vi "Analyze.vi"(8 "error in (no error)":errorcluster, 10 "Image in":T1, 11 "Analyze Q-Factor in":refnum<class "Analyze q-Factor.lvclass">) -> (0 "error out":errorcluster, 1 "Results":refnum<class "Analyze Results Base.lvclass">, 2 "Image out":T1, 3 "Analyze Q-Factor out":refnum<class "Analyze q-Factor.lvclass">)   [LabVIEW 2020, in "Analyze.lvlib" / "Analyze q-Factor.lvclass"]
uses:
  Analyze q-Factor.lvclass
  C:/POLARIS Programme/POLARIS-AS-3-Cams/Submodules/HIJ Vision/Analyze/Analyze Classes/Analyze BaseClass/Analyze BaseClass/Analyze BaseClass.lvclass
  <vilib>/vision/Image Controls.llb/IMAQ Image.ctl
  Results and Overlays/Results Base/Analyze Results Base.lvclass
  Results and Overlays/Results q-Factor/Analyze Results q-Factor.lvclass
  C:/POLARIS Programme/POLARIS-AS-3-Cams/Submodules/HIJ Vision/Analyze/Results and Overlays/Results Base/Analyze Results Base.lvclass
  Results and Overlays/Results Fluence/Analyze Results Fluence.lvclass
  Analyze Parameter/Analyze Parameter Width Method/Width Method.lvclass
  C:/POLARIS Programme/POLARIS-AS-3-Cams/Submodules/HIJ Vision/Analyze/Analyze Parameter/Analyze Parameter Base/Analyze Parameter Base.lvclass
  Results and Overlays/Results q-Factor/Analyze Results q-Factor.lvclass/Analyze Results q-Factor.ctl
  Results and Overlays/Results q-Factor/Write A.vi
  Results and Overlays/Results q-Factor/Write q.vi
  Results and Overlays/Results q-Factor/Write Focus ROI.vi
  Results and Overlays/Results q-Factor/Write Width Method.vi
  Analyze Fluence/Analyze Fluence.lvclass
  <vilib>/vision/NI_Vision_Development_Module.lvlib
  Analyze BaseClass/Analyze BaseClass/Analyze BaseClass.lvclass
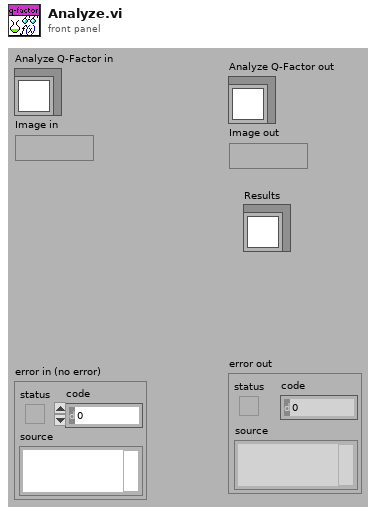
[diagram p1: front panel]
types:
  T1 = typedef "IMAQ Image.ctl" = refnum<image>
  T2 = typedef "Image Type" = u32
  T3 = typedef "Analyze.lvlib/Analyze Fluence.lvclass/Fluence Info.ctl" = cluster{"Fluence J/cm^2":dbl[unit], "Energy in Area":dbl[unit], "max value":i64, "Max fluence area":cluster{"Left":i32, "Top":i32, "Right":i32, "Bottom":i32}}
  T4 = cluster{"Left":i32, "Top":i32, "Right":i32, "Bottom":i32, sgl}
  T5 = typedef "ROI Descriptor" = cluster{"Global Rectangle":i32[], "Contours":cluster{"ID":enum32{"External", "Internal"}, "Type":u32, "Coordinates":i32[]}[]}
  T6 = typedef "POLARIS Vision utility.lvlib/Width Method.ctl" = enum16{"FWHM", "1/e", "1/e^2", "80%", "90%"}
  T7 = cluster{"Mean Value":sgl, "Standard Variation":sgl, "Minimal Value":sgl, "Maximal Value":sgl, "Area (calibrated)":sgl, "Area (pixels)":i32, "%":sgl}
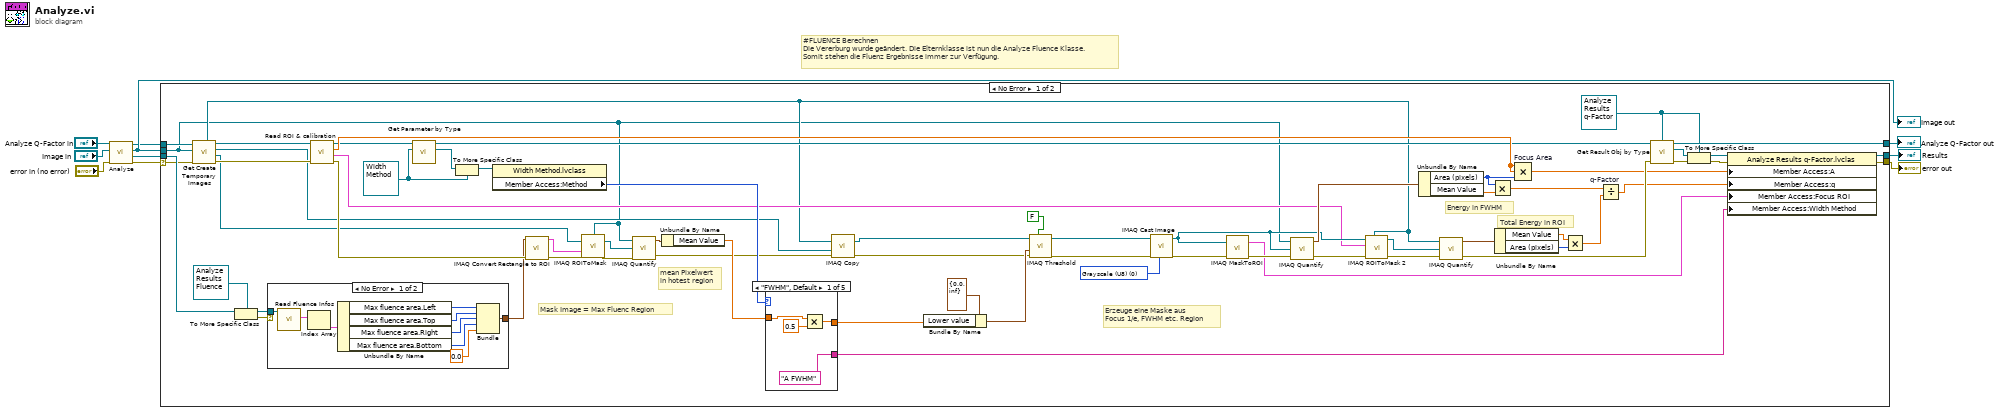
[diagram p0: block diagram]
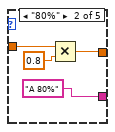
[diagram p3: hidden frame]
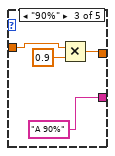
[diagram p4: hidden frame]
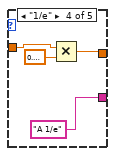
[diagram p5: hidden frame]
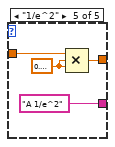
[diagram p6: hidden frame]
diagram:
  # "#FLUENCE Berechnen\nDie Vererburg wurde geändert. Die Elternklasse ist nun die Analyze Fluence Klasse.\nSomit stehen die Fluenz Ergebnisse immer zur Verfügung."
  n1 = call-parent "Analyze.vi"("error in (no error)"="error in (no error)", "Image in"="Image in", "Analyze Fluence in"="Analyze Q-Factor in") -> ("error out"=w2:errorcluster, "Result"=w4:refnum<class "Analyze Results Base.lvclass">, "Image out"=w10:T1, "Analyze Fluence out"=w6:refnum<class "Analyze q-Factor.lvclass">)  [unwired: 5 in]
  "Image out" <- w10
  n2 = case shown="No Error" w2 {
    selector: w2 -> [w21 w106]
    tunnel: w10 -> [w11 _]
    tunnel: w6 -> [w49 w107]
    tunnel: [w44 w105] -> w5
    tunnel: w4 -> [w36 w105]
    tunnel: [w27 w107] -> w3
    tunnel: [w43 w106] -> w1
    frame No Error {
      w29 = refnum<class "Width Method.lvclass"> refnum ("Width Method.lvclass")
      w24 = refnum<class "Analyze Results q-Factor.lvclass"> refnum ("Analyze Results q-Factor.lvclass")
      w70 = T2 0 items=["Grayscale (U8)", "Grayscale (I16)", "Grayscale (SGL)", "Complex (CSG)", "RGB (U32)", "HSL (U32)", "RGB (U64)", "Grayscale (U16)"] ("Image Type")
      # "Erzeuge eine Maske aus \nFocus 1/e, FWHM etc. Region"
      # "Mask Image = Max Fluenc Region"
      # "mean Pixelwert\nin hotest region"
      # "Total Energy in ROI"
      # "Energy in FWHM"
      n3 = call-dynamic "Get Create Temporary Images.vi"("error in (no error)"=w21, "Image in"=w11, "Analyze BaseClass in"=w49) -> ("error out"=w52:errorcluster, "image mask"=w18:T1, "work image"=w32:T1, "Analyze BaseClass out"=w68:refnum<class "Analyze q-Factor.lvclass">, "masked image"=w12:T1)  [unwired: 4 in]
      n4 = To More Specific Class(target class=refnum<class "Analyze Results Fluence.lvclass"> refnum ("Analyze Results Fluence.lvclass"), reference=w36) -> (specific class reference=w35:refnum<class "Analyze Results Fluence.lvclass">, error out=w33:errorcluster)  [unwired: 1 in]
      n5 = case shown="No Error" w33 {
        tunnel: [w83 _] -> w42
        tunnel: w35 -> [w76 _]
        frame No Error {
          n6 = call-dynamic "Read Fluence Infos.vi"("Analyze Results Fluence in"=w76) -> ("Fluence Infos"=w78:T3[])  [unwired: 8 in, 2 out]
          n7 = Index Array(array=w78) -> (element=w77:T3)  [unwired: 1 in]
          n8 = Unbundle By Name(w77) -> ("Max fluence area.Left"=w82:i32, "Max fluence area.Top"=w81:i32, "Max fluence area.Right"=w80:i32, "Max fluence area.Bottom"=w79:i32)
          n9 = Bundle("Left"=w82, "Top"=w81, "Right"=w80, "Bottom"=w79, sgl 0.0) -> (w83:T4)  [unwired: 1 in]
        }
        frame Error {
        }
      }
      n10 = call-dynamic "Read ROI & calibration.vi"("error in (no error)"=w52, "Analyze BaseClass in"=w68) -> ("error out"=w51:errorcluster, "ROI Descriptor"=w14:T5, "calibration mm/px"=w61:dbl[unit], "Analyze BaseClass out"=w37:refnum<class "Analyze q-Factor.lvclass">)  [unwired: 6 in]
      n11 = call "Get Parameter by Type.vi"("Parameter Type"=w29, "Analyze BaseClass in"=w37) -> ("Parameter"=w30:refnum<class "Analyze Parameter Base.lvclass">, "Analyze BaseClass out"=w31:refnum<class "Analyze q-Factor.lvclass">)  [unwired: 6 in, 2 out]
      n12 = To More Specific Class(target class=w29, reference=w30) -> (specific class reference=w28:refnum<class "Width Method.lvclass">)  [unwired: 1 in, 1 out]
      n13 = property class="Width Method.lvclass"(reference=w28) -> ("Member Access:Method"=w50:T6)  [unwired: 1 in, 2 out]
      n14 = call "IMAQ Convert Rectangle to ROI"("error in (no error)"=w51, "Rectangle"=w42) -> ("error out"=w40:errorcluster, "ROI Descriptor"=w41:T5)  [unwired: 7 in]
      n15 = call "IMAQ ROIToMask"("error in (no error)"=w40, "ROI Descriptor"=w41, "Image"=w18, "Image Model"=w11) -> ("error out"=w39:errorcluster, "Image Out"=w56:T1)  [unwired: 2 in, 1 out]
      n16 = call "IMAQ Quantify"("error in (no error)"=w39, "Image Mask"=w56, "Image"=w11) -> ("error out"=w20:errorcluster, "Global Report"=w38:T7)  [unwired: 1 out]
      n17 = Unbundle By Name(w38) -> ("Mean Value"=w55:sgl)
      n18 = case shown="\"FWHM\", Default" w50 {
        tunnel: w55 -> [w87 w91 w95 w99 w104]
        tunnel: [w86 w90 w94 w98 w103] -> w62
        tunnel: ["A FWHM" "A 80%" "A 90%" "A 1/e" "A 1/e^2"] -> w47
        frame "FWHM", Default {
          n19 = Multiply(x=w87, y=0.5) -> (x*y=w86:dbl)
        }
        frame "80%" {
          n20 = Multiply(x=w91, y=0.8) -> (x*y=w90:dbl)
        }
        frame "90%" {
          n21 = Multiply(x=w95, y=0.9) -> (x*y=w94:dbl)
        }
        frame "1/e" {
          n22 = Multiply(x=w99, y=0.36787944117144233) -> (x*y=w98:dbl)
        }
        frame "1/e^2" {
          w102 = 0.36787944117144233
          n23 = Compound Arithmetic op=MULTIPLY(w104, w102, w102) -> (w103:dbl)
        }
      }
      n24 = call "IMAQ Copy"("error in (no error)"=w20, "Image Dst"=w32, "Image Src"=w12) -> ("error out"=w19:errorcluster, "Image Dst Out"=w17:T1)  [unwired: 3 in]
      n25 = Bundle By Name(cluster=cluster{"Lower value":sgl, "Upper value":sgl} {"Lower value"=0.0, "Upper value"=inf} ("Range"), "Lower value"=w62) -> (w73:cluster{"Lower value":sgl, "Upper value":sgl})
      n26 = call "IMAQ Threshold"("Keep/Replace Value (Replace)"=FALSE, "error in (no error)"=w19, "Range"=w73, "Image Src"=w17) -> ("error out"=w71:errorcluster, "Image Dst Out"=w72:T1)  [unwired: 6 in]
      n27 = call "IMAQ Cast Image"("Image Type"=w70, "error in (no error)"=w71, "Image Src"=w72) -> ("error out"=w58:errorcluster, "Image Dst Out"=w15:T1)  [unwired: 7 in]
      n28 = call "IMAQ MaskToROI"("Image"=w15, "error in (no error)"=w58) -> ("ROI Descriptor"=w46:T5, "error out"=w57:errorcluster)  [unwired: 5 in, 1 out]
      n29 = call "IMAQ Quantify"("error in (no error)"=w57, "Image Mask"=w15, "Image"=w11) -> ("error out"=w53:errorcluster, "Global Report"=w69:T7)  [unwired: 1 out]
      n30 = call "IMAQ ROIToMask 2"("Image Model"=w12, "error in (no error)"=w53, "ROI Descriptor"=w14, "Image"=w15) -> ("error out"=w16:errorcluster, "Image Out"=w13:T1)  [unwired: 5 in, 1 out]
      n31 = Unbundle By Name(w69) -> ("Area (pixels)"=w59:i32, "Mean Value"=w60:sgl)
      n32 = call "IMAQ Quantify"("error in (no error)"=w16, "Image Mask"=w13, "Image"=w12) -> ("error out"=w75:errorcluster, "Global Report"=w65:T7)  [unwired: 1 out]
      n33 = Multiply(x=w59, y=w60) -> (x*y=w63:sgl)
      n34 = Unbundle By Name(w65) -> ("Mean Value"=w67:sgl, "Area (pixels)"=w66:i32)
      n35 = Compound Arithmetic op=MULTIPLY "Focus Area"(w61, w61, w59) -> (w45:dbl[unit])
      n36 = Multiply(x=w67, y=w66) -> (x*y=w64:sgl)
      n37 = Divide "q-Factor"(x=w63, y=w64) -> (x/y=w48:sgl)
      n38 = call "Get Result Obj by Type.vi"("error in (no error)"=w75, "Parameter Type"=w24, "Analyze BaseClass in"=w31) -> ("error out"=w26:errorcluster, "Parameter"=w25:refnum<class "Analyze Results Base.lvclass">, "Analyze BaseClass out"=w27:refnum<class "Analyze q-Factor.lvclass">)  [unwired: 5 in, 1 out]
      n39 = To More Specific Class(target class=w24, reference=w25, error in=w26) -> (specific class reference=w23:refnum<class "Analyze Results q-Factor.lvclass">, error out=w22:errorcluster)
      n40 = property class="Analyze Results q-Factor.lvclas"(reference=w23, error in=w22, "Member Access:A"=w45, "Member Access:q"=w48, "Member Access:Focus ROI"=w46, "Member Access:Width Method"=w47) -> (reference out=w44:refnum<class "Analyze Results q-Factor.lvclass">, error out=w43:errorcluster)
    }
    frame Error {
    }
  }
  "error out" <- w1
  "Analyze Q-Factor out" <- w3
  "Results" <- w5
